vi "Get Data Log File Settings.vi"(8 "error in":errorcluster, 10 "Target Type":T1, 11 "File Ref in":T2 format="%.0x") -> (0 "error out":errorcluster, 1 "Timestamp":bool, 2 "File Path":path, 3 "File Ref out":T2 format="%.0x", 4 "Archive Files":bool, 5 "Name":string, 6 "Log Archive Directory":path)   [LabVIEW 2018, in "Embedded Data Logger System Explorer.lvlib"]
uses:
  Embedded Data Logger System Explorer.lvlib
  <vilib>/NI Veristand/Custom Device API/Custom Device Item Ref.ctl
  <vilib>/NI Veristand/Custom Device API/Custom Device Target Type.ctl
  Shared/Constants.vi
  <vilib>/NI Veristand/Custom Device API/Get Item Property (String Array).vi
  <vilib>/NI Veristand/Custom Device API/Get Item Property (Boolean).vi
  <vilib>/NI Veristand/Custom Device API/Custom Device API.lvlib
  Shared/Embedded Data Logger Shared.lvlib
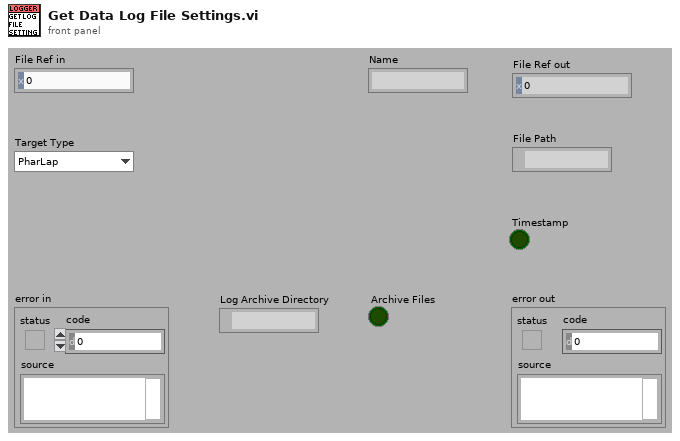
[diagram p1: front panel]
types:
  T1 = typedef "Custom Device API.lvlib/Custom Device Target Type.ctl" = enum16{"PharLap", "VxWorks", "Windows", "Linux_32_ARM", "Linux_x64"}
  T2 = typedef "Custom Device API.lvlib/Custom Device Item Ref.ctl" = u64
  T3 = typedef "Custom Device API.lvlib/Custom Device Item Info.ctl" = cluster{"Name":string, "Is Channel":bool, "GUID":string, "Is Waveform":bool}
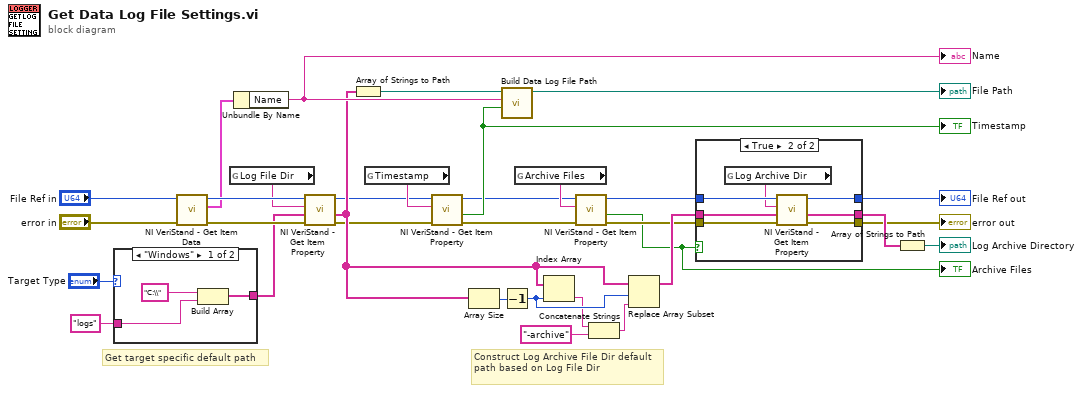
[diagram p0: block diagram]
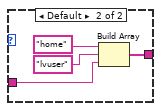
[diagram p3: hidden frame]
diagram:
  # "Construct Log Archive File Dir default path based on Log File Dir"
  # "Get target specific default path"
  n1 = case shown="\"Windows\"" "Target Type" {
    tunnel: [w34 w37] -> w22
    tunnel: "logs" -> [w35 w38]
    frame "Windows" {
      n2 = Build Array("C:\\", w35) -> (w34:string[])
    }
    frame Default {
      n3 = Build Array("home", "lvuser", w38) -> (w37:string[])
    }
  }
  n4 = call <vilib>:"NI VeriStand - Get Item Data.vi"("error in (no error)"="error in", "Item Ref in"="File Ref in") -> ("error out"=w32:errorcluster, "Item Info"=w28:T3, "Item Ref out"=w33:T2)  [unwired: 7 out]
  n5 = global read "Constants.vi" "Log File Dir"() -> (w9:string)
  n6 = Unbundle By Name(w28) -> ("Name"=w30:string)
  "Name" <- w30
  n7 = call-poly <vilib>:"NI VeriStand - Get Item Property.vi"("error in (no error)"=w32, "Default Value"=w22, "Property Name"=w9, "Item Ref in"=w33) -> ("error out"=w3:errorcluster, "Value"=w15:string[], "Item Ref out"=w4:T2)  [unwired: 5 out]
  n8 = Array of Strings to Path(0:w15) -> (2:w21:path)  [unwired: 1 in]
  n9 = global read "Constants.vi" "Timestamp"() -> (w7:string)
  n10 = call-poly <vilib>:"NI VeriStand - Get Item Property.vi"("error in (no error)"=w3, "Property Name"=w7, "Item Ref in"=w4) -> ("error out"=w1:errorcluster, "Value"=w29:bool, "Item Ref out"=w2:T2)  [unwired: 1 in, 5 out]
  "Timestamp" <- w29
  n11 = Array Size(array=w15) -> (size(s)=w20:i32)
  n12 = call "Build Data Log File Path.vi"("Timestamp"=w29, "Name"=w30, "Log File Directory"=w21) -> ("appended path"=→"File Path":path)  [unwired: 7 in, 1 out]
  n13 = Decrement(x=w20) -> (x-1=w19:i32)
  n14 = global read "Constants.vi" "Archive Files"() -> (w8:string)
  n15 = Index Array(array=w15, index=w19) -> (element=w17:string)
  n16 = call-poly <vilib>:"NI VeriStand - Get Item Property.vi"("error in (no error)"=w1, "Property Name"=w8, "Item Ref in"=w2) -> ("error out"=w11:errorcluster, "Value"=w10:bool, "Item Ref out"=w12:T2)  [unwired: 1 in, 5 out]
  "Archive Files" <- w10
  n17 = Concatenate Strings(w17, "-archive") -> (w16:string)
  n18 = Replace Array Subset(array=w15, new element=w16, index=w19) -> (w14:string[])
  n19 = case shown="True" w10 {
    tunnel: [w43 w50] -> w25
    tunnel: w14 -> [w43 w49]
    tunnel: w12 -> [w41 w48]
    tunnel: [w41 w47] -> w5
    tunnel: w11 -> [w42 w46]
    tunnel: [w42 w45] -> w6
    frame False {
      # "Archive disabled. Base archive directory on Log File Dir"
    }
    frame True {
      n20 = global read "Constants.vi" "Log Archive Dir"() -> (w44:string)
      n21 = call-poly <vilib>:"NI VeriStand - Get Item Property.vi"("error in (no error)"=w46, "Default Value"=w49, "Property Name"=w44, "Item Ref in"=w48) -> ("error out"=w45:errorcluster, "Value"=w50:string[], "Item Ref out"=w47:T2)  [unwired: 5 out]
    }
  }
  "File Ref out" <- w5
  "error out" <- w6
  n22 = Array of Strings to Path(0:w25) -> (2:→"Log Archive Directory":path)  [unwired: 1 in]
